vi "getHighestScore.vi"(8 "error in":errorcluster) -> (0 "error out":errorcluster, 2 "Highest Score Achineved Time":string, 3 "Highest Score":string)   [LabVIEW 2024]
uses:
  session.vi
  <vilib>/httpClient/LabVIEWHTTPClient.lvlib
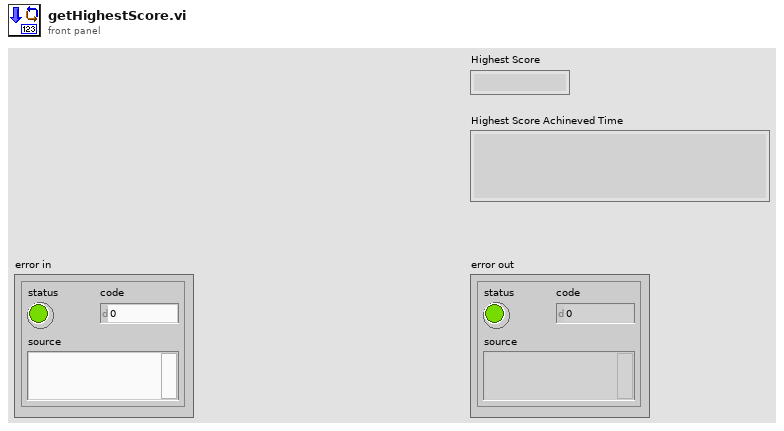
[diagram p1: front panel]
types:
  T1 = typedef "LabVIEWHTTPClient.lvlib/ClientHandle.ctl" = refnum<k1>
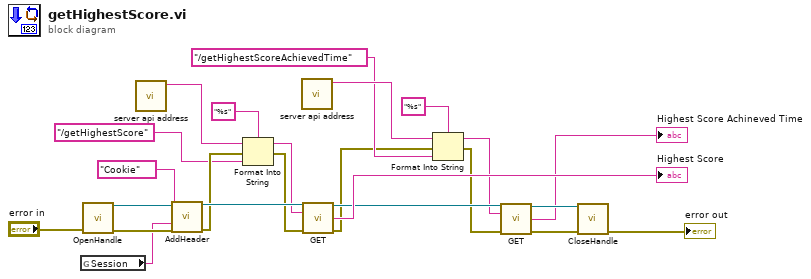
[diagram p0: block diagram]
diagram:
  n1 = global read "session.vi" "Session"() -> (w20:string)
  n2 = call <vilib>:"OpenHandle.vi"("error in (no error)"="error in") -> ("client handle out"=w22:T1, "error out"=w23:errorcluster)  [unwired: 13 in]
  n3 = call "server api address.vi"() -> ("Server API URL"=w15:string)  [unwired: 11 in]
  n4 = call <vilib>:"AddHeader.vi"("client handle"=w22, "header"="Cookie", "value"=w20, "error in (no error)"=w23) -> ("client handle out"=w19:T1, "error out"=w18:errorcluster)  [unwired: 10 in]
  n5 = Format Into String(format string="%s", initial string=w15, error in=w18, "/getHighestScore" ("input 1")) -> (resulting string=w16:string, error out=w17:errorcluster)
  n6 = call "server api address.vi"() -> ("Server API URL"=w10:string)  [unwired: 11 in]
  n7 = call <vilib>:"GET.vi"("client handle"=w19, "url"=w16, "error in (no error)"=w17) -> ("client handle out"=w8:T1, "body"=→"Highest Score":string, "error out"=w6:errorcluster)  [unwired: 9 in, 1 out]
  n8 = Format Into String(format string="%s", initial string=w10, error in=w6, "/getHighestScoreAchievedTime" ("input 1")) -> (resulting string=w4:string, error out=w5:errorcluster)
  n9 = call <vilib>:"GET.vi"("client handle"=w8, "url"=w4, "error in (no error)"=w5) -> ("client handle out"=w3:T1, "body"=→"Highest Score Achineved Time":string, "error out"=w2:errorcluster)  [unwired: 9 in, 1 out]
  n10 = call <vilib>:"CloseHandle.vi"("client handle"=w3, "error in (no error)"=w2) -> ("error out"=→"error out":errorcluster)  [unwired: 13 in]
